vi "Fake DAQ Test.vi"() -> ()   [LabVIEW 2013]
uses:
  lib/DAQ IO/Fake/Interpolate Actions.ctl
  lib/Data Access Objects/Metadata/Persistant DAO Actions.ctl
  lib/DAQ IO/Daq Actions.ctl
  lib/Data Access Objects/Metadata/LBCB Number.ctl
  lib/Data Access Objects/Metadata/LBCB Location.ctl
panel:
  out "Fake Responses":dbl[](array[numeric])
  in  "Number of Steps":i32=500
  in  "OM  Location":T1=enum."Portable LBCB"
  in  "Delay":u32=2
  in  "Log Filename":string="FakeDAQData"
  out "Text Output File":path=path "C:/Documents and Settings/mbletzin/Desktop/Work/Operations Manager/AutobalanceStates.txt"
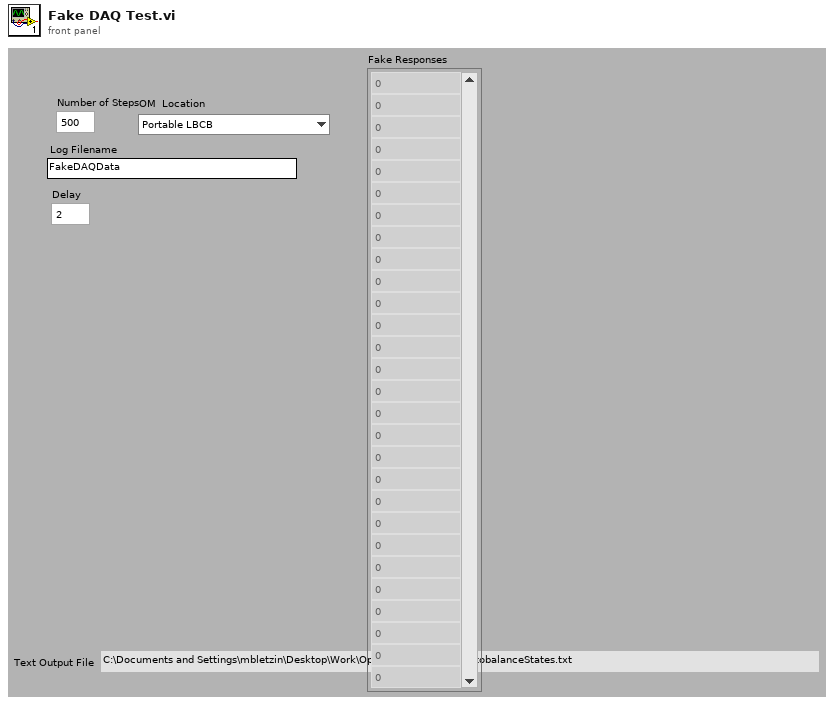
[diagram p1: front panel]
types:
  T1 = typedef "LBCB Location.ctl" = enum16{"Crane Bay Two LBCB", "Crane Bay One LBCB", "5th Scale Two LBCB", "5th Scale One LBCB", "Portable LBCB", "University of Houston LBCB"}
  T2 = enum16{"open", "replace", "create", "open or create", "replace or create", "replace or create with confirmation"}
  T3 = typedef "LBCB Number.ctl" = enum16{"LBCB1", "LBCB2"}
  T4 = typedef "Daq Actions.ctl" = enum16{"Init", "Send Commands", "Get Responses", "Stop"}
  T5 = typedef "Persistant DAO Actions.ctl" = enum16{"Init", "Get", "Set", "Load", "Save"}
  T6 = typedef "Interpolate Actions.ctl" = enum16{"Init", "Interpolate"}
  T7 = typedef "Number Of LBCBs.ctl" = enum16{"1", "2"}
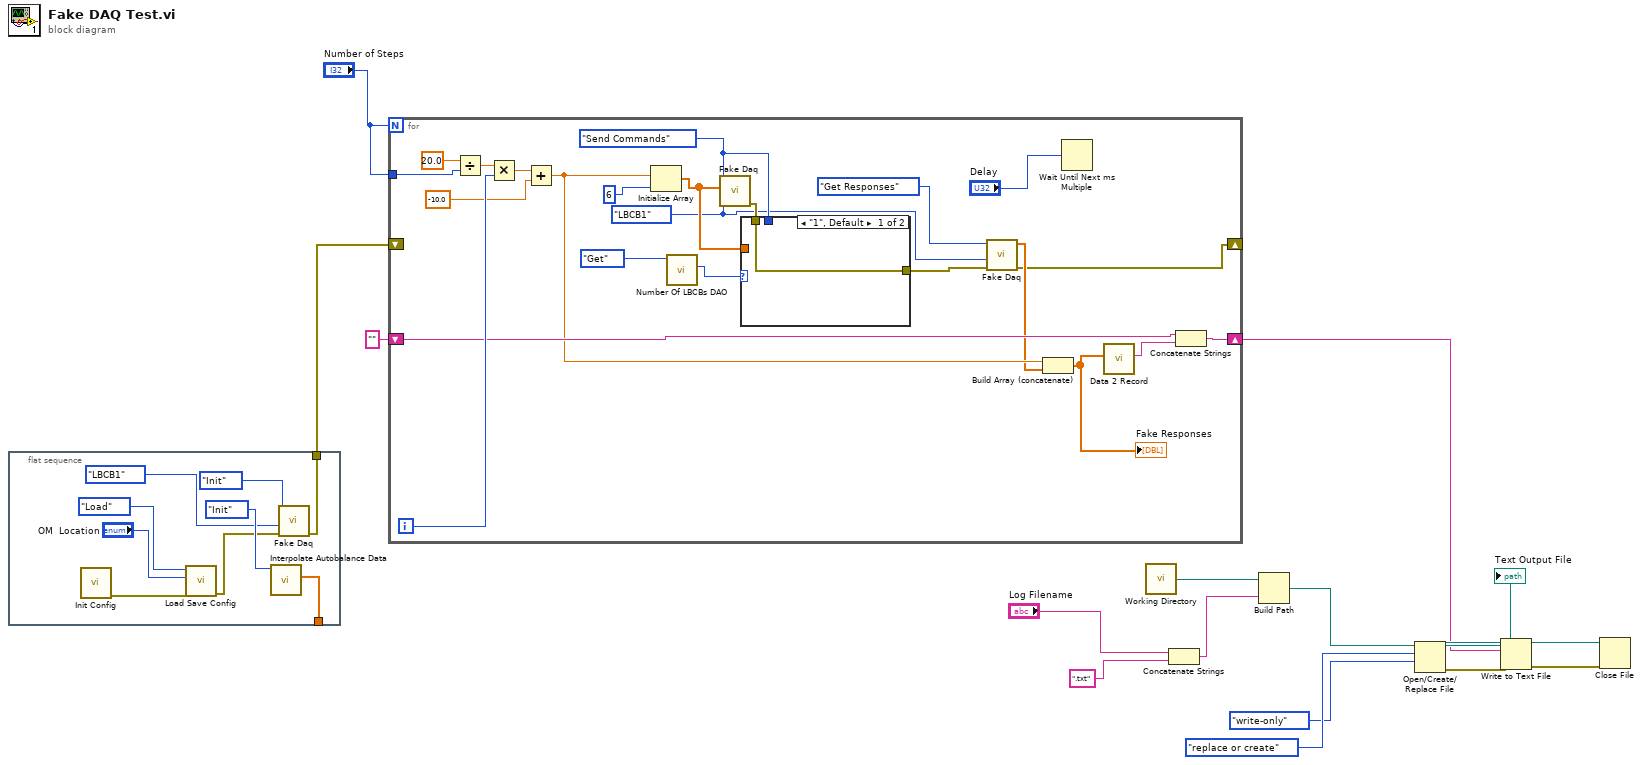
[diagram p0: block diagram]
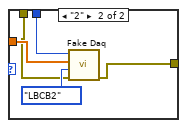
[diagram p2: hidden frame]
diagram:
  n1 = flat-sequence {
    tunnel: [w23] -> _
    tunnel: [w17] -> w2
    frame #0 {
      n2 = call "Init Config.vi"() -> ("error out"=w22:errorcluster)  [unwired: 1 in, 10 out]
      n3 = call "Load Save Config.vi"("error in (no error)"=w22, "OM  Location"="OM  Location", "Actions"=Persistant_DAO_Actions."Load") -> ("error out"=w19:errorcluster)  [unwired: 1 in, 7 out]
      n4 = call "Interpolate Autobalance Data.vi"("Actions"=Interpolate_Actions."Init") -> ("Servo Errors"=w23:dbl[])  [unwired: 3 in, 7 out]
      n5 = call "Fake Daq.vi"("error in (no error)"=w19, "LBCB Number"=LBCB_Number."LBCB1", "Fake Daq Actions"=Daq_Actions."Init") -> ("error out"=w17:errorcluster)  [unwired: 1 in, 7 out]
    }
  }
  n6 = for {
    N: "Number of Steps" -> [_]
    shift-right: [w25] -> _
    shift-left: w2 -> [_]
    shift-right: [w31] -> w4
    shift-left: "" ("Records Out") -> [w32]
    tunnel: "Number of Steps" -> [w45]
    i -> [w43]
    w26 = LBCB_Number."LBCB1" ("LBCB Number")
    w37 = Daq_Actions."Send Commands" ("Fake Daq Actions")
    n7 = Divide(x=20.0, y=w45) -> (x/y=w44:dbl)
    n8 = Multiply(x=w44, y=w43) -> (x*y=w42:dbl)
    n9 = Add(x=w42, y=-10.0) -> (x+y=w29:dbl)
    n10 = Initialize Array(w29, 6 ("dimension size")) -> (w36:dbl[])
    n11 = call "Number Of LBCBs DAO.vi"("Actions"=Persistant_DAO_Actions."Get") -> ("Number of\nLBCBs Out"=w38:T7)  [unwired: 3 in, 7 out]
    n12 = call "Fake Daq.vi"("LBCB Number"=w26, "Commands"=w36, "Fake Daq Actions"=w37) -> ("error out"=w35:errorcluster)  [unwired: 1 in, 7 out]
    n13 = case shown="\"1\", Default" w38 {
      tunnel: w37 -> [_ w53]
      tunnel: w36 -> [_ w52]
      tunnel: w35 -> [w48 w50]
      tunnel: [w48 w49] -> w34
      frame "1", Default {
      }
      frame "2" {
        n14 = call "Fake Daq.vi"("error in (no error)"=w50, "LBCB Number"=LBCB_Number."LBCB2", "Commands"=w52, "Fake Daq Actions"=w53) -> ("error out"=w49:errorcluster)  [unwired: 7 out]
      }
    }
    n15 = call "Fake Daq.vi"("error in (no error)"=w34, "LBCB Number"=w26, "Fake Daq Actions"=Daq_Actions."Get Responses") -> ("error out"=w25:errorcluster, "Responses"=w28:dbl[])  [unwired: 1 in, 6 out]
    n16 = Build Array (concatenate)(w29, w28) -> (w27:dbl[])
    "Fake Responses" <- w27
    n17 = Wait Until Next ms Multiple(millisecond multiple="Delay") -> ()  [unwired: 1 out]
    n18 = call "Data 2 Record.vi"("Data"=w27) -> ("Records"=w30:string)  [unwired: 2 in, 8 out]
    n19 = Concatenate Strings(w32, w30) -> (w31:string)
  }
  n20 = call "Working Directory.vi"() -> ("Path"=w8:path)  [unwired: 1 out]
  n21 = Concatenate Strings("Log Filename", ".txt" ("string")) -> (w9:string)
  n22 = Build Path(base path=w8, name or relative path=w9) -> (appended path=w7:path)
  "Text Output File" <- w7
  n23 = Open/Create/Replace File(file path (use dialog)=w7, operation (0:open)=T2."replace or create", access (0:read/write)=enum16{"read/write", "read-only", "write-only"}."write-only") -> (refnum out=w12:refnum<file>, error out=w13:errorcluster)  [unwired: 1 in, 3 out]
  n24 = Write to Text File(file (use dialog)=w12, text=w4, error in=w13) -> (refnum out=w14:refnum<file>, error out=w15:errorcluster)  [unwired: 2 out]
  n25 = Close File(refnum=w14, error in=w15) -> ()  [unwired: 2 out]
